vi "Read.vi"(8 "error in (no error)":errorcluster, 11 "Double Float.lvclass in":refnum<class "Subtract_Time-Time.lvclass">) -> (0 "error out":errorcluster, 2 "Value":dbl, 3 "Double Float.lvclass out":refnum<class "Subtract_Time-Time.lvclass">)   [LabVIEW 2021, in "Subtract_Time-Time.lvclass"]
uses:
  Subtract_Time-Time.lvclass
  Subtract_Time-Time.lvclass/Subtract_Time-Time.ctl
  Abs_Types/Time/Abs_Time.lvclass
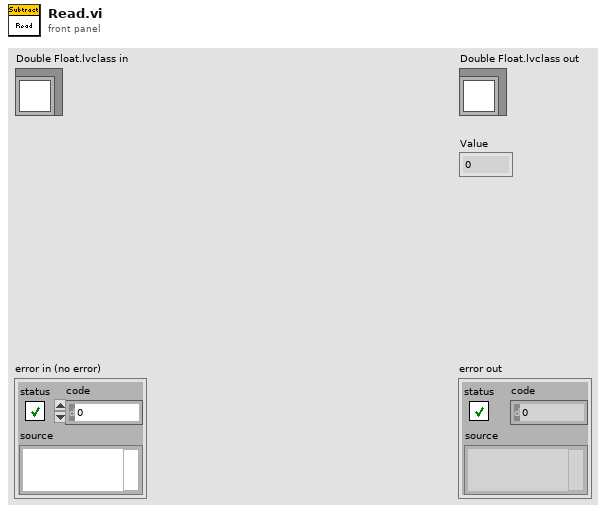
[diagram p1: front panel]
types:
  T1 = typedef "Abs_Time.lvclass/Type.ctl" = timestamp
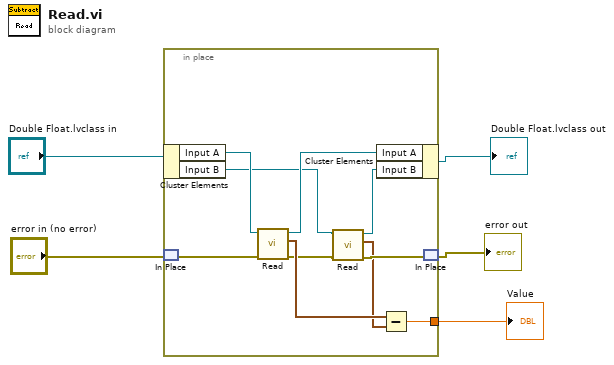
[diagram p0: block diagram]
diagram:
  n1 = in-place {
    in-place-border: [w11] -> w1
    n2 = in-place-cluster #1("Double Float.lvclass in") -> ("Input A"=w15:refnum<class "Abs_Time.lvclass">, "Input B"=w10:refnum<class "Abs_Time.lvclass">)
    n3 = in-place-match #2("error in (no error)") -> (w13:errorcluster)
    n4 = call-dynamic "Read.vi"("error in (no error)"=w13, "Double Float.lvclass_340760 in"=w15) -> ("error out"=w8:errorcluster, "Value"=w12:T1, "Double Float.lvclass_340760 out"=w14:refnum<class "Abs_Time.lvclass">)  [unwired: 7 in]
    n5 = call-dynamic "Read.vi"("error in (no error)"=w8, "Double Float.lvclass_340760 in"=w10) -> ("error out"=w7:errorcluster, "Value"=w6:T1, "Double Float.lvclass_340760 out"=w9:refnum<class "Abs_Time.lvclass">)  [unwired: 7 in]
    n6 = in-place-cluster #1("Input A"=w14, "Input B"=w9) -> (→"Double Float.lvclass out":refnum<class "Subtract_Time-Time.lvclass">)
    n7 = Subtract(x=w12, y=w6) -> (x-y=w11:dbl)
    n8 = in-place-match #2(w7) -> (→"error out":errorcluster)
  }
  "Value" <- w1
